vi "Арифметический блок.vi"(2 "c":T1, 3 "c-1":bool, 4 "b":bool, 5 "a":bool) -> (0 "c":bool, 1 "s":bool)   [LabVIEW 2013]
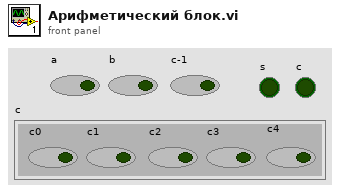
[diagram p1: front panel]
types:
  T1 = cluster{"c0":bool, "c1":bool, "c2":bool, "c3":bool, "c4\nc4":bool}
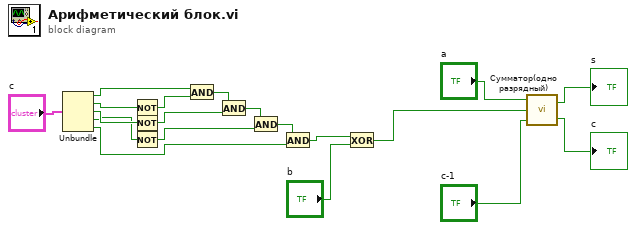
[diagram p0: block diagram]
diagram:
  n1 = Unbundle("c") -> ("c0"=w10:bool, "c1"=w9:bool, "c2"=w8:bool, "c3"=w7:bool, "c4\nc4"=w3:bool)
  n2 = Not(x=w9) -> (.not. x?=w16:bool)
  n3 = Not(x=w8) -> (.not. x?=w15:bool)
  n4 = Not(x=w7) -> (.not. x?=w14:bool)
  n5 = And(x=w10, y=w16) -> (x .and. y?=w11:bool)
  n6 = And(x=w11, y=w15) -> (x .and. y?=w12:bool)
  n7 = And(x=w12, y=w14) -> (x .and. y?=w13:bool)
  n8 = And(x=w13, y=w3) -> (x .and. y?=w6:bool)
  n9 = Exclusive Or(1:"b", 2:w6) -> (0:w4:bool)
  n10 = call "Сумматор(одноразрядный).vi"("c-1"="c-1", "b"=w4, "a"="a") -> ("c"=→"c":bool, "s"=→"s":bool)
